vi "Test Get Terminal Name.vi"() -> ()   [LabVIEW 2014]
uses:
  <vilib>/DAQmx/create/channels.llb/DAQmx Create Channel (DO-Digital Output).vi
  <resource>/objmgr/daqmx.rc
panel:
  out "Terminals":tag[](array[tag])
  out "PhysicalChanName":tag
  out "Terminal Name with Device Prefix":tag
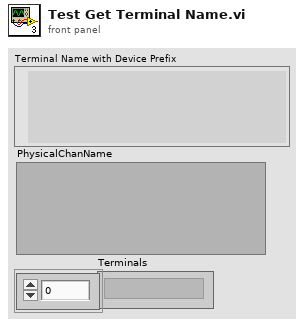
[diagram p1: front panel]
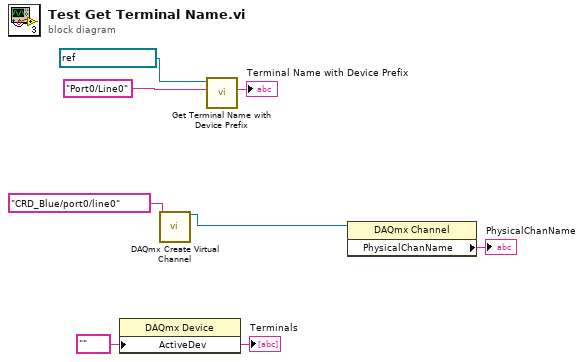
[diagram p0: block diagram]
diagram:
  w2 = tag "" ("ActiveDev")
  n1 = property class="DAQmx Device"("ActiveDev"=w2) -> ()  [unwired: 2 in, 2 out]
  n2 = call-poly <vilib>:"DAQmx Create Virtual Channel.vi"("lines"=tag "CRD_Blue/port0/line0") -> ("task out"=w4:refnum<k21>)  [unwired: 13 in, 1 out]
  n3 = call "Get Terminal Name with Device Prefix.vi"("Local Terminal Name"="Port0/Line0", "task/channels in"=refnum<k21> "CRDS Blue AI") -> ("Terminal Name with Device Prefix"=→"Terminal Name with Device Prefix":tag)  [unwired: 7 in, 2 out]
  n4 = property class="DAQmx Channel"(reference=w4) -> ("PhysicalChanName"=→"PhysicalChanName":tag)  [unwired: 1 in, 2 out]
  "Terminals" <- w2
